vi "LogCheckError.vi"(8 "Msg":string, 11 "error in (no error)":errorcluster) -> ()   [LabVIEW 2011]
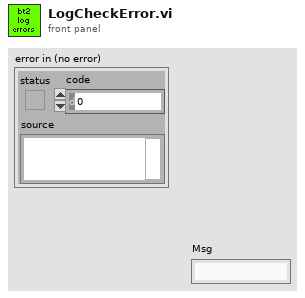
[diagram p1: front panel]
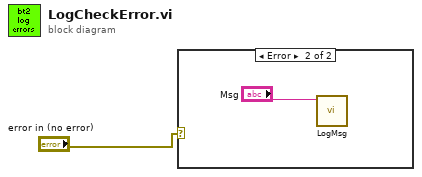
[diagram p0: block diagram]
diagram:
  n1 = case shown="Error" "error in (no error)" {
    frame No Error {
    }
    frame Error {
      n2 = call "LogMsg.vi"("msg"="Msg") -> ()  [unwired: 11 in]
    }
  }
